vi "Constants.vi"() -> ()   [LabVIEW 2020, in "AIM MIL-STD-1553 Shared.lvlib"]
doc: "Use this Global VI to access the GUIDs assigned to the page resources of the Custom Device."
uses:
  AIM MIL-STD-1553 Shared.lvlib
panel:
  in  "Tab Control":enum32{"GUIDs", "Constants", "Properties"}(tab)=enum."Constants"
  in  "RTM Wrapper":string="2631586A-EF3F-4497-A632-0D1C06305D5E"
  in  "Compiled.Settings":string="Compiled.Settings"
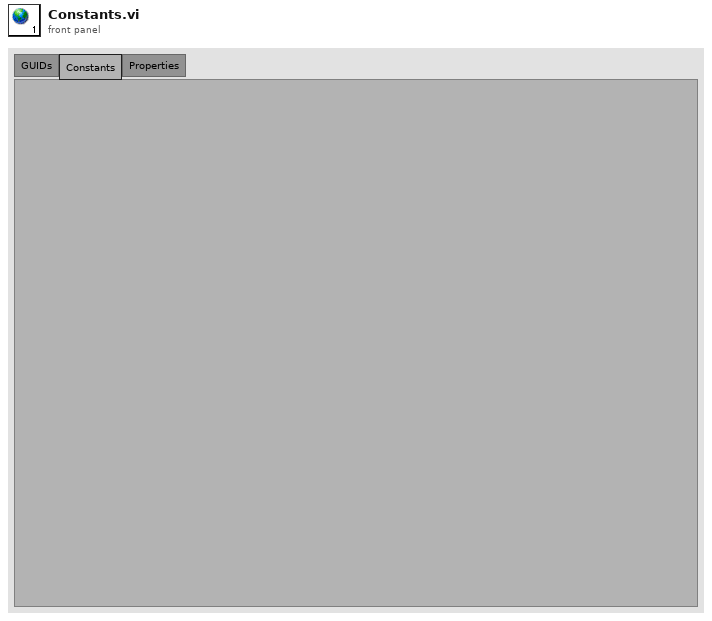
[diagram p1: front panel]
diagram:
